vi "MeasurementService Editor Constants.vi"() -> (3 "Measurement Helpers":string="Measurement Helpers")   [LabVIEW 2020, in "MeasurementService Editor.lvlib"]
doc: "Holds the string constants for the Measurement Service Editor library."
uses:
  MeasurementService Editor.lvlib
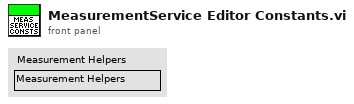
[diagram p1: front panel]
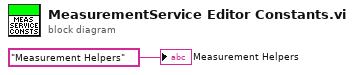
[diagram p0: block diagram]
diagram:
  "Measurement Helpers" <- "Measurement Helpers" ("Measurement Helpers")
